vi "Set Domain.vi"(8 "error in (no error)":errorcluster, 10 "domain":variant, 11 "Domain_Steady_2D_Polygon in":refnum<class "NI_Domain_Steady_2D_Polygon.lvclass">) -> (0 "error out":errorcluster, 3 "Domain_Steady_2D_Polygon out":refnum<class "NI_Domain_Steady_2D_Polygon.lvclass">)   [LabVIEW 2020, in "NI_PDE.lvlib" / "NI_Domain_Steady_2D_Polygon.lvclass"]
uses:
  <vilib>/gmath/pde.llb/DomainClass/Domain_Steady_2D_Polygon/NI_Domain_Steady_2D_Polygon.lvclass
  <vilib>/gmath/pde.llb/DomainClass/Domain_Steady_2D_Polygon/Domain Data.ctl
  <vilib>/gmath/pde.llb/DomainClass/Domain_Steady_2D_Polygon/NI_Domain_Steady_2D_Polygon.lvclass/NI_Domain_Steady_2D_Polygon.ctl
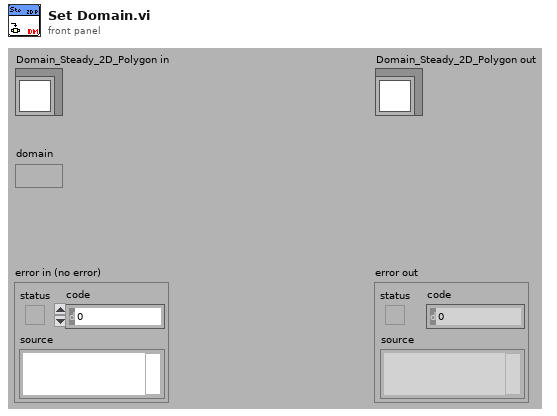
[diagram p1: front panel]
types:
  T1 = typedef "NI_PDE.lvlib/NI_Domain_Steady_2D_Polygon.lvclass/Domain Data.ctl" = cluster{"X":dbl[], "Y":dbl[], "Xi":dbl[], "Yi":dbl[], "grid factor":dbl, "Triangulation":i32[][]}
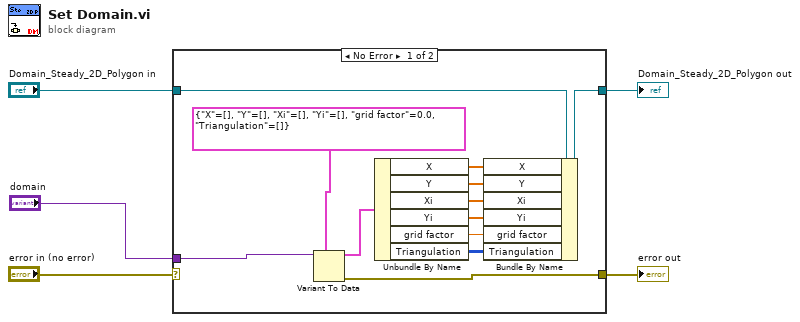
[diagram p0: block diagram]
diagram:
  n1 = case shown="No Error" "error in (no error)" {
    selector: "error in (no error)" -> [_ w19]
    tunnel: "Domain_Steady_2D_Polygon in" -> [w14 w18]
    tunnel: [w13 w18] -> w5
    tunnel: [w12 w19] -> w4
    tunnel: "domain" -> [w17 _]
    frame No Error {
      n2 = Variant To Data(type=T1 {"X"=[], "Y"=[], "Xi"=[], "Yi"=[], "grid factor"=0.0, "Triangulation"=[]} ("domain data"), Variant=w17) -> (data=w16:T1, error out=w12:errorcluster)  [unwired: 1 in]
      n3 = Unbundle By Name(w16) -> ("X"=w11:dbl[], "Y"=w10:dbl[], "Xi"=w9:dbl[], "Yi"=w8:dbl[], "grid factor"=w7:dbl, "Triangulation"=w6:i32[][])
      n4 = Bundle By Name(cluster=w14, "X"=w11, "Y"=w10, "Xi"=w9, "Yi"=w8, "grid factor"=w7, "Triangulation"=w6) -> (w13:refnum<class "NI_Domain_Steady_2D_Polygon.lvclass">)
    }
    frame Error {
    }
  }
  "Domain_Steady_2D_Polygon out" <- w5
  "error out" <- w4
